vi "str to uint16.vi"(2 "String":string) -> (6 "uint16":u16)   [LabVIEW 2014, in "OPCUA XML.lvlib"]
uses:
  OPCUA XML.lvlib
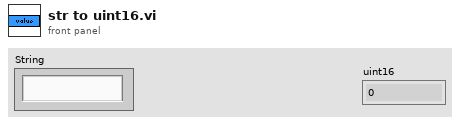
[diagram p1: front panel]
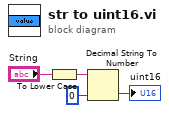
[diagram p0: block diagram]
diagram:
  n1 = To Lower Case(string="String") -> (all lower case string=w3:string)
  n2 = Decimal String To Number(string=w3, default (0L)=u16 0 ("default (0 I32)")) -> (number=→"uint16":u16)  [unwired: 1 in, 1 out]
